vi "Ctor.vi"(8 "error in (no error)":errorcluster, 11 "Endpoint in":refnum<class "Endpoint.lvclass">) -> (0 "error out":errorcluster, 3 "Endpoint out":refnum<class "Endpoint.lvclass">)   [LabVIEW 2020, in "Stream.lvlib" / "Endpoint.lvclass"]
uses:
  Endpoint.lvclass
  URI/URI.lvclass
  State Callback.ctl
  Ref Data.ctl
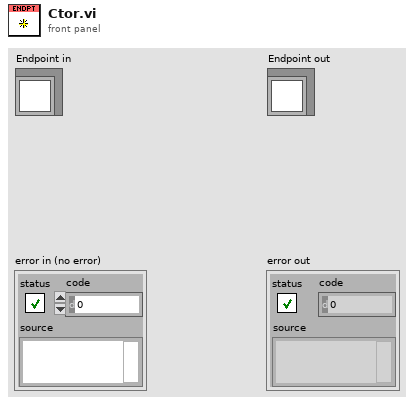
[diagram p1: front panel]
types:
  T1 = typedef "Stream.lvlib/Endpoint.lvclass/Ref Data.ctl" = cluster{"URI":refnum<class "URI.lvclass">, "State Callbacks":T2[], "Sniffer Callbacks":T2[]}
  T2 = typedef "Stream.lvlib/Endpoint.lvclass/State Callback.ctl" = cluster{"Owner":refnum<class>, "VI":refnum<vi>, "Context":variant}
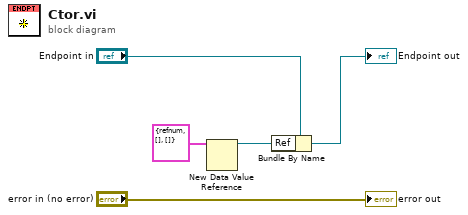
[diagram p0: block diagram]
diagram:
  n1 = New Data Value Reference(data value=T1 {"URI"=refnum, "State Callbacks"=[], "Sniffer Callbacks"=[]} ("Ref Data")) -> (data value reference=w2:refnum<data-value>)  [unwired: 1 in, 1 out]
  n2 = Bundle By Name(cluster="Endpoint in", "Ref"=w2) -> (→"Endpoint out":refnum<class "Endpoint.lvclass">)
  "error out" <- "error in (no error)"
